vi "Test 1.vi"(8 "error in (no error)":errorcluster, 11 "Test Case In":refnum<class "Tests.lvclass">) -> (0 "error out":errorcluster, 3 "Test Case Out":refnum<class "Tests.lvclass">)   [LabVIEW 2020, in "Tests.lvclass"]
uses:
  Tests.lvclass
  Tests.lvclass/Tests.ctl
  4993e8ee-a06a-463a-9684-69129f64d5ce.vi
  Proto/Proto.lvclass
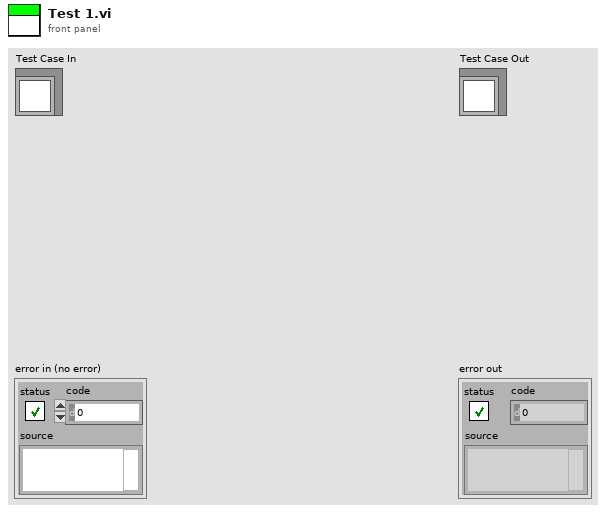
[diagram p1: front panel]
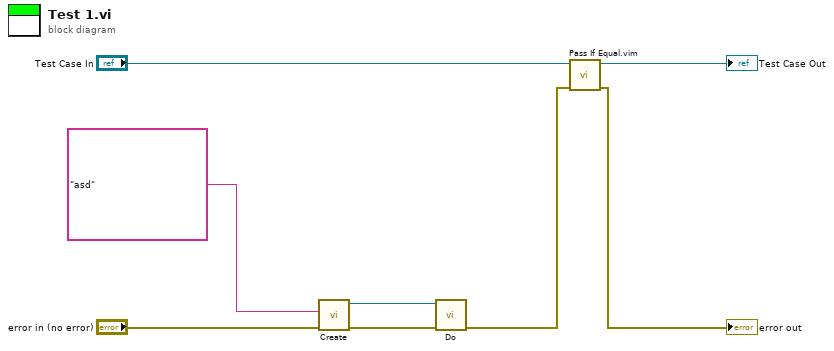
[diagram p0: block diagram]
diagram:
  n1 = call "Create.vi"("error in (no error)"="error in (no error)", "Input"="asd") -> ("error out"=w4:errorcluster, "Proto"=w2:refnum<class "Proto.lvclass">)  [unwired: 8 in]
  n2 = call "Do.vi"("error in (no error)"=w4, "Proto in"=w2) -> ("error out"=w3:errorcluster)  [unwired: 8 in, 1 out]
  n3 = call "Pass If Equal.vim"("error in (no error)"=w3, "LUnit Test Case In"="Test Case In") -> ("error out"=→"error out":errorcluster, "LUnit Test Case Out"=→"Test Case Out":refnum<class "Tests.lvclass">)  [unwired: 8 in]
